vi "rounding_number.vi"(9 "power of ten":dbl format="%#_15g", 10 "Array":dbl[](array[numeric])) -> (2 "rounded":dbl[](array[numeric]))   [LabVIEW 2019]
doc: "LabVIEW only readily supports rounding numbers to integer values. For example, LabVIEW rounds the number 543.21 to 543.00.\n\nThis VI shows how to round numbers to values other than integers. For example, you can round the number 543.21 to 543.20 or 540.00 by choosing which decimal place you want to round to."
panel:
  out "Decimal place":dbl=1.0 format="%#_9f"
  # "Select Help»Show Context Help and move the cursor over the VI icon to display help for this VI."
  # "Instructions:\n1. Run the VI.\n2. Enter a number you want to round.\n3. Enter a power of ten to select which decimal place to round to.\n4. Repeat steps 2 and 3 until you no longer want to round numbers.\n5. Click the Stop button to stop the VI."
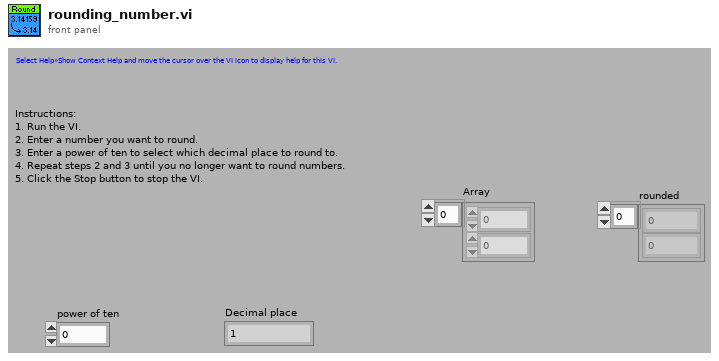
[diagram p1: front panel]
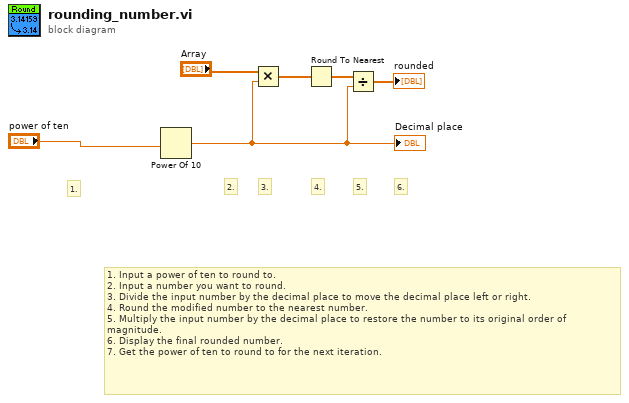
[diagram p0: block diagram]
diagram:
  # "6."
  # "5."
  # "4."
  # "3."
  # "2."
  # "1."
  # "1. Input a power of ten to round to.\n2. Input a number you want to round.\n3. Divide the input number by the decimal place to move the decimal place left or right.\n4. Round the modified number to the nearest number.\n5. Multiply the input number by the decimal place to restore the number to its original order of magnitude.\n6. Display the final rounded number.\n7. Get the power of ten to round to for the next iteration."
  n1 = Power Of 10(x="power of ten") -> (10^x=w4:dbl)
  "Decimal place" <- w4
  n2 = Multiply(x="Array", y=w4) -> (x*y=w6:dbl[])
  n3 = Round To Nearest(number=w6) -> (nearest integer value=w5:dbl[])
  n4 = Divide(x=w5, y=w4) -> (x/y=→"rounded":dbl[])
